vi "Main.vi"(11 "Module Admin":refnum<class "Delacor_lib_QMH_Cloneable Module Admin.lvclass">) -> ()   [LabVIEW 2025, in "USB IO.lvlib"]
doc: "This template is based off of the Queued Message Handler design pattern and the Queued Message Handler project template that ships with LabVIEW.\n\nThe main difference is that the queue is private to this module and communication between modules is performed via Broadcast and Request events.\n\nRequest events are wrapped in public API methods and are handled in the Event Handling Loop (EHL) of this VI. Any module can register for Broadcast events sent by this module. The EHL generates messages based on user interface actions.\n\nThe Message Handling Loop (MHL) processes messages generated by the EHL, or by other messages. The messages are string values, so new messages can be added easily to the Message Cases case structure in the MHL. Each message cluster can also provide an optional value for Message Data, which is a variant that can be converted to whatever message-specific data is required.\n_____\nBased on DQMH Dev Tools: Project Template 7.1.2.1547."
uses:
  USB IO.lvlib
  <vilib>/Delacor/Delacor QMH/Libraries/Message Queue_class/Delacor_lib_QMH_Message Queue.lvclass
  Module Data--cluster.ctl
  <vilib>/Utility/miscctls.llb/LVPointTypeDef.ctl
  <vilib>/Delacor/Delacor QMH/Libraries/Message Queue_class/Delacor_lib_QMH_Enqueue Message (Single).vi
  Stop Argument--cluster.ctl
  <vilib>/Delacor/Delacor QMH/Libraries/Cloneable Module Admin_class/Delacor_lib_QMH_Cloneable Module Admin.lvclass
  Display Lines (Reply Payload)--cluster.ctl
  Display Lines Argument--cluster.ctl
  Classes/USB IO generic/USB IO.lvclass
  select child (Reply Payload)--cluster.ctl
  Classes/Hardware Selection.ctl
  select child Argument--cluster.ctl
  Classes/Arduino Uno/Arduino Uno.lvclass
  Classes/USB-6000/USB-6000.lvclass
  read config (Reply Payload)--cluster.ctl
  read config Argument--cluster.ctl
  init device (Reply Payload)--cluster.ctl
  init device Argument--cluster.ctl
  stop device (Reply Payload)--cluster.ctl
  stop device Argument--cluster.ctl
  Controls/Numeric Voltage.ctl
  analog read (Reply Payload)--cluster.ctl
  analog read Argument--cluster.ctl
  digital write (Reply Payload)--cluster.ctl
  digital write Argument--cluster.ctl
  reconnect (Reply Payload)--cluster.ctl
  reconnect Argument--cluster.ctl
  C:/Users/grove/Desktop/LabVIEW/Git/atp-station/Libraries/USB IO/Classes/USB IO generic/USB IO.lvclass
  C:/Users/grove/Desktop/LabVIEW/Git/atp-station/Libraries/USB IO/Classes/USB-6000/USB-6000.lvclass
  C:/Users/grove/Desktop/LabVIEW/Git/atp-station/Libraries/USB IO/Classes/Arduino Uno/Arduino Uno.lvclass
panel:
  out "error out":errorcluster
  out "Status":string
  in  "Simulate EHL Error":bool
  in  "Simulate MHL Error":bool
  # "Other processes communicate with this Module via its Public API (wrappers for its Request Events).\n\nThis Module communicates with other processes via its Broadcast Events.\nAny process that wants to receive these messages can register for this module's Broadcast events."
  # "This template is for the DQMH framework. See the block diagram for more information on how to use this template."
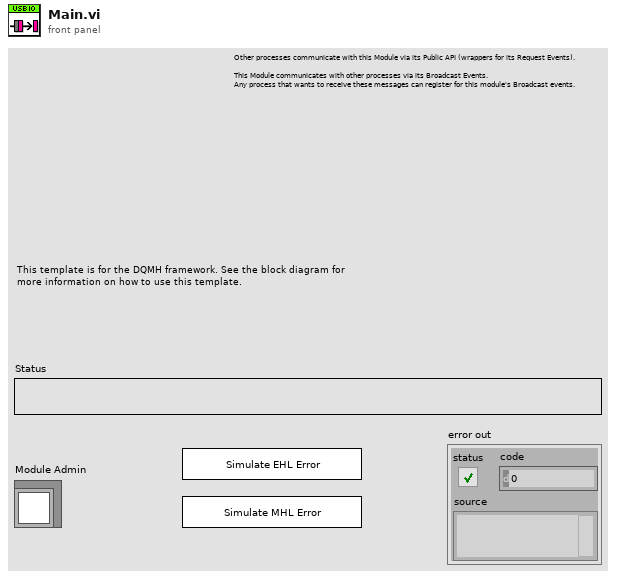
[diagram p1: front panel]
types:
  T1 = typedef "USB IO.lvlib/Request Events--cluster.ctl" = cluster{"Stop Module":refnum<user-event>, "Show Panel":refnum<user-event>, "Hide Panel":refnum<user-event>, "Show Diagram":refnum<user-event>, "Get Module Execution Status":refnum<user-event>, "Display Lines":refnum<user-event>, "select child":refnum<user-event>, "read config":refnum<user-event>, "init":refnum<user-event>, "init device":refnum<user-event>, "stop device":refnum<user-event>, "analog read":refnum<user-event>, "digital write":refnum<user-event>, "reconnect":refnum<user-event>}
  T2 = typedef "USB IO.lvlib/Module Data--cluster.ctl" = cluster{"Status":string, "USB IO.lvlib:USB IO.lvclass":refnum<class "USB IO.lvclass">}
  T3 = enum32{"invalid lock state", "Not Locked", "Locked (No Password)", "Password-protected"}
  T4 = typedef "USB IO.lvlib/Stop Argument--cluster.ctl" = cluster{"Module ID":i32, "Origin":string, "Exit via Stop Module Req?":bool, "Wait for Module to stop?":bool}
  T5 = typedef "USB IO.lvlib/Display Lines Argument--cluster.ctl" = cluster{"Module ID":i32, "Wait Notifier":refnum<notifier>, "wait for reply":bool}
  T6 = typedef "USB IO.lvlib/select child Argument--cluster.ctl" = cluster{"Module ID":i32, "Hardware":T7, "Wait Notifier":refnum<notifier>, "wait for reply":bool}
  T7 = typedef "Hardware Selection.ctl" = enum16{"Simulation", "USB-6000", "USB-6001", "Arduino Uno"}
  T8 = typedef "USB IO.lvlib/read config Argument--cluster.ctl" = cluster{"Module ID":i32, "Path":path, "Wait Notifier":refnum<notifier>, "wait for reply":bool}
  T9 = typedef "USB IO.lvlib/init device Argument--cluster.ctl" = cluster{"Module ID":i32, "Variant":variant, "Wait Notifier":refnum<notifier>, "wait for reply":bool}
  T10 = typedef "USB IO.lvlib/stop device Argument--cluster.ctl" = cluster{"Module ID":i32, "Wait Notifier":refnum<notifier>, "wait for reply":bool}
  T11 = typedef "USB IO.lvlib/analog read Argument--cluster.ctl" = cluster{"Module ID":i32, "Line":string, "Wait Notifier":refnum<notifier>, "wait for reply":bool}
  T12 = typedef "USB IO.lvlib/digital write Argument--cluster.ctl" = cluster{"Module ID":i32, "Line":string, "On/Off":bool, "Wait Notifier":refnum<notifier>, "wait for reply":bool}
  T13 = typedef "USB IO.lvlib/reconnect Argument--cluster.ctl" = cluster{"Module ID":i32, "Wait Notifier":refnum<notifier>, "wait for reply":bool}
  T14 = typedef "LVPointTypeDef.ctl" = cluster{"Horizontal":i16, "Vertical":i16}
  T15 = enum32{"Invalid", "Standard", "Closed", "Hidden", "Minimized", "Maximized"}
  T16 = typedef "USB IO.lvlib/Display Lines (Reply Payload)--cluster.ctl" = cluster{"Module ID":i32, "Lines":string[], "Values":i32[], "error":errorcluster}
  T17 = typedef "USB IO.lvlib/select child (Reply Payload)--cluster.ctl" = cluster{"Module ID":i32, "error":errorcluster}
  T18 = typedef "USB IO.lvlib/read config (Reply Payload)--cluster.ctl" = cluster{"Module ID":i32, "error":errorcluster}
  T19 = typedef "USB IO.lvlib/init device (Reply Payload)--cluster.ctl" = cluster{"Module ID":i32, "error":errorcluster}
  T20 = typedef "USB IO.lvlib/stop device (Reply Payload)--cluster.ctl" = cluster{"Module ID":i32, "error":errorcluster}
  T21 = typedef "USB IO.lvlib/analog read (Reply Payload)--cluster.ctl" = cluster{"Module ID":i32, "Voltage":T22, "error":errorcluster}
  T22 = typedef "Numeric Voltage.ctl" = dbl
  T23 = typedef "USB IO.lvlib/digital write (Reply Payload)--cluster.ctl" = cluster{"Module ID":i32, "error":errorcluster}
  T24 = typedef "USB IO.lvlib/reconnect (Reply Payload)--cluster.ctl" = cluster{"Module ID":i32, "error":errorcluster}
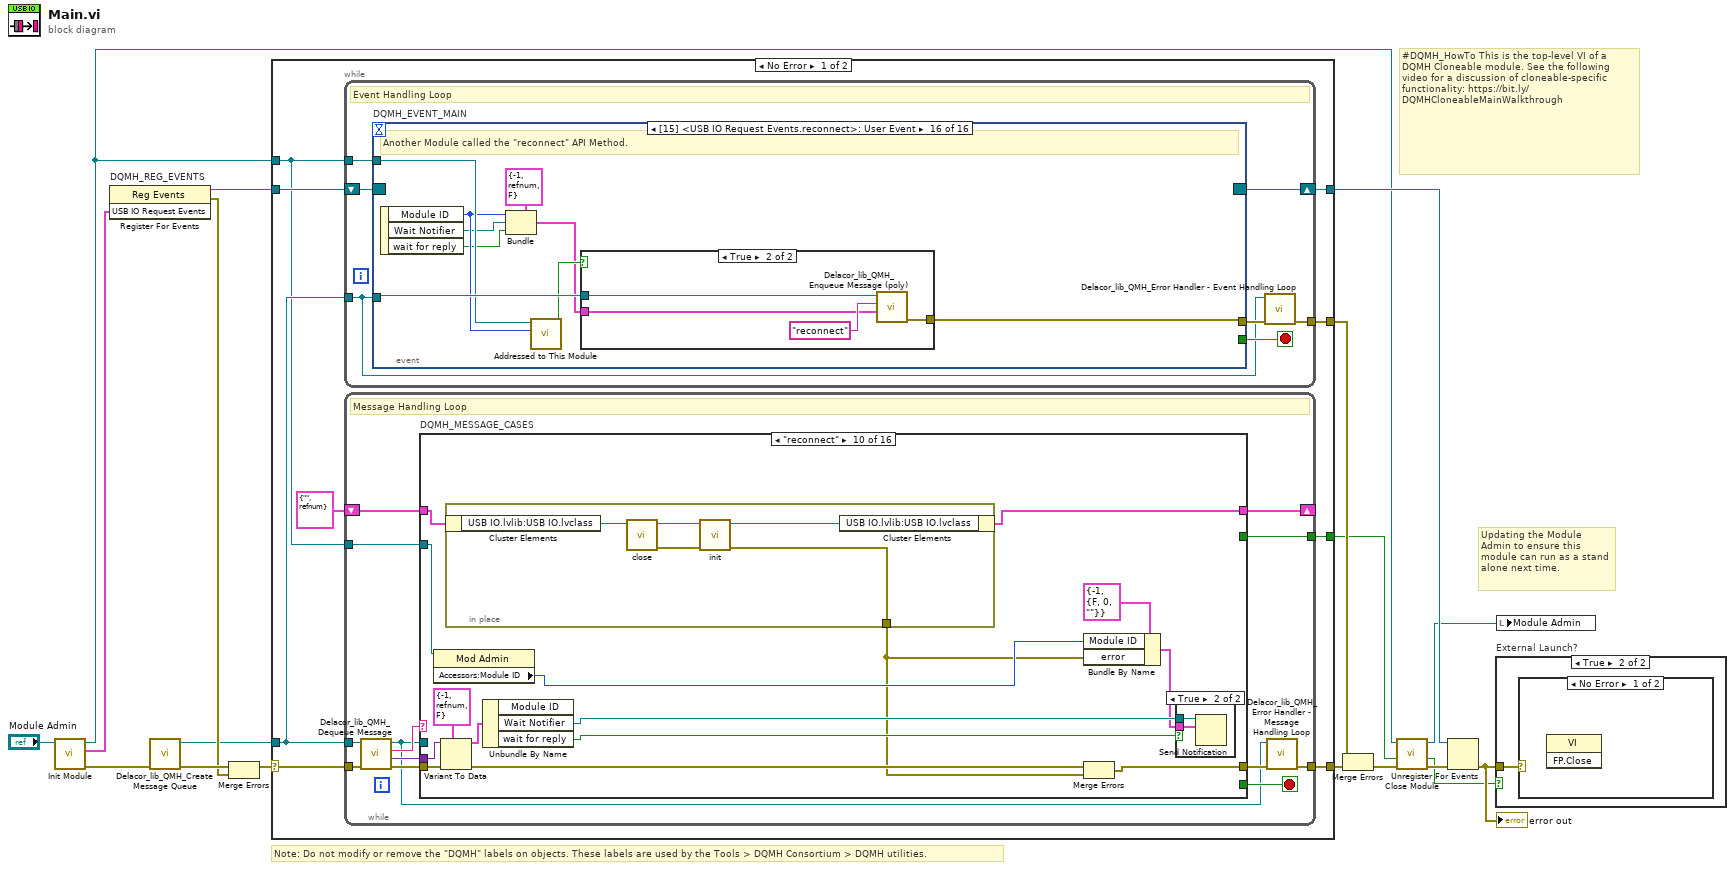
[diagram p0: block diagram]
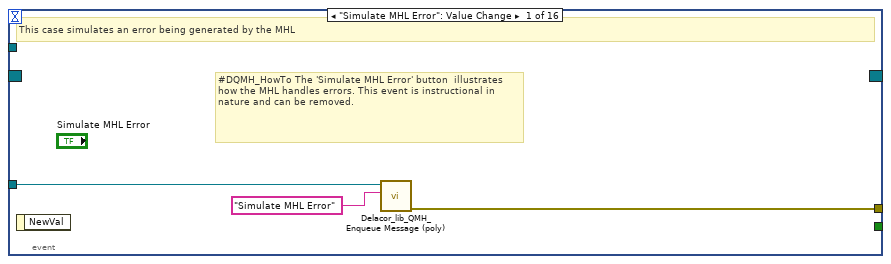
[diagram p2: hidden frame]
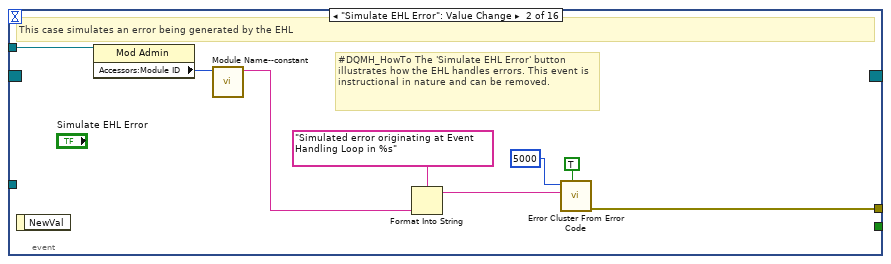
[diagram p3: hidden frame]
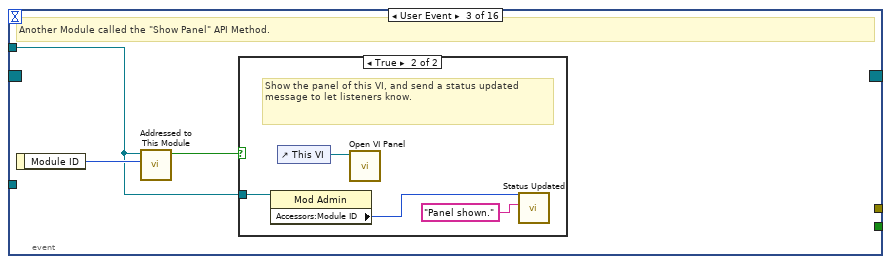
[diagram p4: hidden frame]
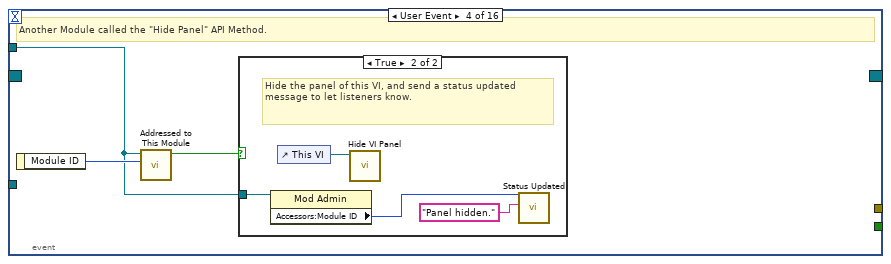
[diagram p6: hidden frame]
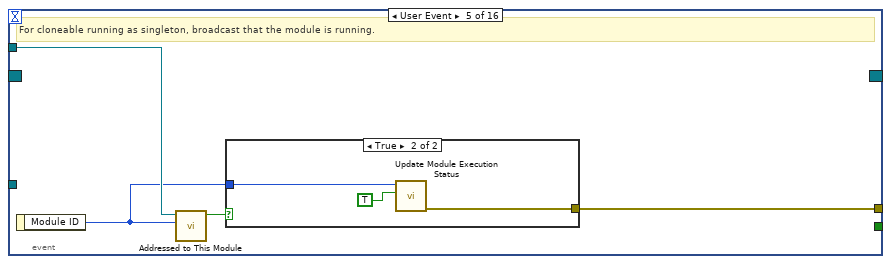
[diagram p8: hidden frame]
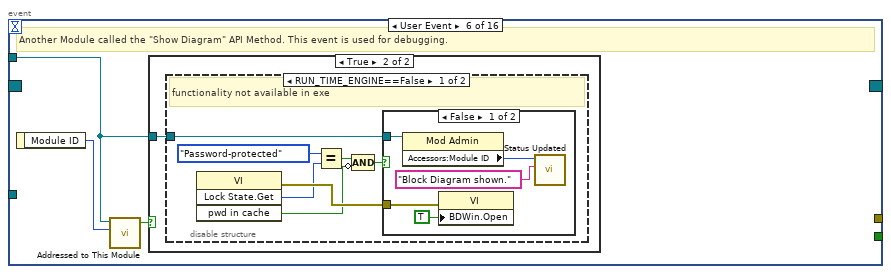
[diagram p10: hidden frame]
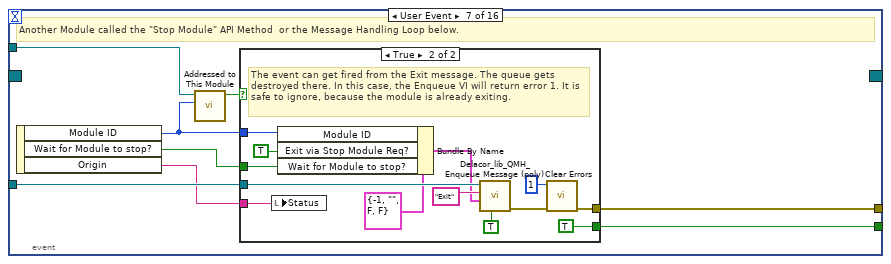
[diagram p14: hidden frame]
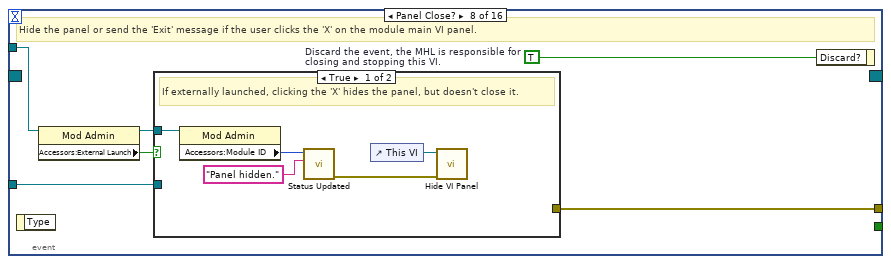
[diagram p16: hidden frame]
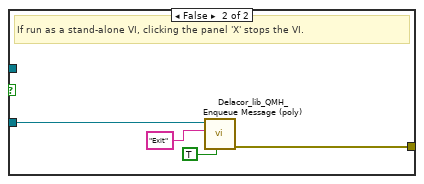
[diagram p17: hidden frame]
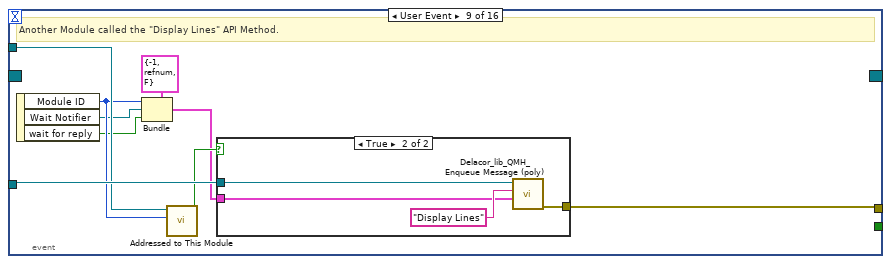
[diagram p18: hidden frame]
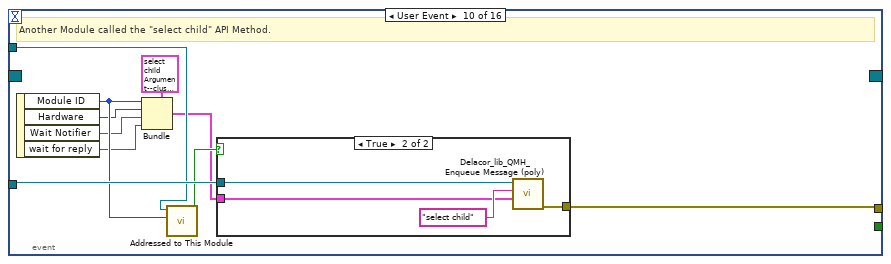
[diagram p20: hidden frame]
diagram:
  # "#DQMH_HowTo This is the top-level VI of a DQMH Cloneable module. See the following video for a discussion of cloneable-specific functionality: https://bit.ly/DQMHCloneableMainWalkthrough"
  # "Note: Do not modify or remove the \"DQMH\" labels on objects. These labels are used by the Tools > DQMH Consortium > DQMH utilities."
  # "Updating the Module Admin to ensure this module can run as a stand alone next time."
  n1 = call "Init Module.vi"("Cloneable Module Admin in"="Module Admin") -> ("error out"=w15:errorcluster, "USB IO Request Events"=w7:T1, "Cloneable Module Admin out"=w4:refnum<class "Delacor_lib_QMH_Cloneable Module Admin.lvclass">)  [unwired: 8 in]
  n2 = register-events "DQMH_REG_EVENTS"(w7) -> (reference out=w8:refnum<event-registration>, error out=w10:errorcluster)  [unwired: 2 in]
  n3 = call <vilib>:"Delacor_lib_QMH_Create Message Queue.vi"("error in"=w15) -> ("error out"=w12:errorcluster, "Message Queue"=w6:refnum<class "Delacor_lib_QMH_Message Queue.lvclass">)  [unwired: 9 in]
  n4 = Merge Errors(w12, w10) -> (w11:errorcluster)
  n5 = case shown="No Error" w11 {
    selector: w11 -> [w25 w517]
    tunnel: [w27 w516] -> w16
    tunnel: [w24 w515] -> w9
    tunnel: w8 -> [w22 w515]
    tunnel: w6 -> [w21 w508]
    tunnel: [w26 _] -> w17
    tunnel: w4 -> [w20 w511]
    tunnel: [w19 _] -> w2
    frame No Error {
      n6 = while {
        tunnel: w21 -> [w28]
        shift-right: [w31] -> w24
        shift-left: w22 -> [w32]
        tunnel: [w33] -> w26
        tunnel: w20 -> [w29]
        stop <- w30 stop-if-true
        # "Event Handling Loop"
        n7 = event "DQMH_EVENT_MAIN" shown="[15] <USB IO Request Events.reconnect>: User Event" {
          selector: w32 -> [_ _ _ _ _ _ _ _ _ _ _ _ _ _ _ _]
          dyn-events: [_ _ _ _ _ _ _ _ _ _ _ _ _ _ _ _] -> w31
          timeout: _ -> [_ _ _ _ _ _ _ _ _ _ _ _ _ _ _ _]
          tunnel: [_ _ _ _ _ _ w86 _ _ _ _ _ _ _ _ _] -> w30
          tunnel: w28 -> [w36 _ _ _ _ _ w89 w106 w127 w141 w155 w169 w182 w196 w211 w224]
          tunnel: [w37 w45 _ _ w63 _ w90 w109 w119 w132 w146 w160 w174 w187 w201 w216] -> w34
          tunnel: w29 -> [_ w44 w46 w53 w61 w67 w88 w107 w125 w139 w153 w167 w180 w194 w209 w222]
          event "Simulate MHL Error": Value Change {
            # "#DQMH_HowTo The 'Simulate MHL Error' button  illustrates how the MHL handles errors. This event is instructional in nature and can be removed."
            # "This case simulates an error being generated by the MHL"
            n8 = event-data() -> ()  [unwired: 1 in, 1 out]
            n9 = call-poly <vilib>:"Delacor_lib_QMH_Enqueue Message (poly).vi"("Message"="Simulate MHL Error", "Message Queue in"=w36) -> ("error out"=w37:errorcluster)  [unwired: 8 in, 1 out]
          }
          event "Simulate EHL Error": Value Change {
            # "#DQMH_HowTo The 'Simulate EHL Error' button  illustrates how the EHL handles errors. This event is instructional in nature and can be removed."
            # "This case simulates an error being generated by the EHL"
            n10 = event-data() -> ()  [unwired: 1 in, 1 out]
            n11 = property on="Property Node" class="Mod Admin"(reference=w44) -> ("Accessors:Module ID"=w43:i32)  [unwired: 1 in, 2 out]
            n12 = call "Module Name--constant.vi"("Module ID"=w43) -> ("Module Name"=w38:string)  [unwired: 10 in]
            n13 = Format Into String(format string="Simulated error originating at Event Handling Loop in %s", w38) -> (resulting string=w41:string)  [unwired: 2 in, 1 out]
            n14 = call <vilib>:"Error Cluster From Error Code.vi"("show call chain? (False)"=TRUE, "error message (\"\")"=w41, "error code (0)"=5000) -> ("error out"=w45:errorcluster)  [unwired: 6 in]
          }
          event User Event {
            # "Another Module called the \"Show Panel\" API Method."
            n15 = event-data() -> ("Module ID"=w47:i32)  [unwired: 1 in]
            n16 = call "Addressed to This Module.vi"("Module ID from Argument"=w47, "Module Admin"=w46) -> ("Addressed to this instance?"=w48:bool)  [unwired: 8 in, 1 out]
            n17 = case shown="True" w48 {
              tunnel: w46 -> [_ w50]
              frame False {
              }
              frame True {
                # "Show the panel of this VI, and send a status updated message to let listeners know."
                n18 = property on="Property Node" class="Mod Admin"(reference=w50) -> ("Accessors:Module ID"=w49:i32)  [unwired: 1 in, 2 out]
                n19 = control-ref of="This VI"() -> (w52:refnum<vi>)
                n20 = call "Open VI Panel.vi"("VI"=w52) -> ()  [unwired: 10 in, 1 out]
                n21 = call "Status Updated.vi"("Status"="Panel shown." ("format string"), "Module ID"=w49) -> ()  [unwired: 9 in, 1 out]
              }
            }
          }
          event User Event {
            # "Another Module called the \"Hide Panel\" API Method."
            n22 = event-data() -> ("Module ID"=w54:i32)  [unwired: 1 in]
            n23 = call "Addressed to This Module.vi"("Module ID from Argument"=w54, "Module Admin"=w53) -> ("Addressed to this instance?"=w55:bool)  [unwired: 8 in, 1 out]
            n24 = case shown="True" w55 {
              tunnel: w53 -> [_ w57]
              frame False {
              }
              frame True {
                # "Hide the panel of this VI, and send a status updated message to let listeners know."
                n25 = property on="Property Node" class="Mod Admin"(reference=w57) -> ("Accessors:Module ID"=w56:i32)  [unwired: 1 in, 2 out]
                n26 = control-ref of="This VI"() -> (w59:refnum<vi>)
                n27 = call "Hide VI Panel.vi"("VI"=w59) -> ()  [unwired: 10 in, 1 out]
                n28 = call "Status Updated.vi"("Status"="Panel hidden." ("format string"), "Module ID"=w56) -> ()  [unwired: 9 in, 1 out]
              }
            }
          }
          event User Event {
            # "For cloneable running as singleton, broadcast that the module is running."
            n29 = event-data() -> ("Module ID"=w60:i32)  [unwired: 1 in]
            n30 = call "Addressed to This Module.vi"("Module ID from Argument"=w60, "Module Admin"=w61) -> ("Addressed to this instance?"=w62:bool)  [unwired: 8 in, 1 out]
            n31 = case shown="True" w62 {
              tunnel: [_ w66] -> w63
              tunnel: w60 -> [_ w65]
              frame False {
              }
              frame True {
                n32 = call "Update Module Execution Status.vi"("Running?"=TRUE, "Module ID"=w65) -> ("error out"=w66:errorcluster)  [unwired: 9 in]
              }
            }
          }
          event User Event {
            # "Another Module called the \"Show Diagram\" API Method. This event is used for debugging."
            n33 = event-data() -> ("Module ID"=w68:i32)  [unwired: 1 in]
            n34 = call "Addressed to This Module.vi"("Module ID from Argument"=w68, "Module Admin"=w67) -> ("Addressed to this instance?"=w69:bool)  [unwired: 8 in, 1 out]
            n35 = case shown="True" w69 {
              tunnel: w67 -> [_ w70]
              frame False {
              }
              frame True {
                n36 = disable-structure shown="RUN_TIME_ENGINE==False" {
                  disable-tunnel: w70 -> [w71 _]
                  frame condition #0 (active) {
                    # "functionality not available in exe"
                    n37 = invoke on="Invoke Node" class="VI" method="Lock State.Get"() -> (error out=w77:errorcluster, "Get Lock State"=w76:T3, "pwd in cache"=w73:bool)  [unwired: 4 in, 1 out]
                    n38 = Equal?(x=T3."Password-protected", y=w76) -> (x = y?=w74:bool)
                    n39 = Compound Arithmetic op=AND(w74, invert w73) -> (w72:bool)
                    n40 = case shown="False" w72 {
                      tunnel: w77 -> [w82 _]
                      tunnel: w71 -> [w79 _]
                      frame False {
                        n41 = property on="Property Node" class="Mod Admin"(reference=w79) -> ("Accessors:Module ID"=w78:i32)  [unwired: 1 in, 2 out]
                        n42 = property on="Property Node" class="VI"(error in=w82, "BDWin.Open"=TRUE ("Block Diagram Window:Open")) -> ()  [unwired: 1 in, 2 out]
                        n43 = call "Status Updated.vi"("Status"="Block Diagram shown." ("format string"), "Module ID"=w78) -> ()  [unwired: 9 in, 1 out]
                      }
                      frame True {
                        # "Password-protected VI, and the password is not in the cache. Do not show the diagram."
                      }
                    }
                  }
                  frame condition #1 {
                  }
                }
              }
            }
          }
          event User Event {
            # "Another Module called the \"Stop Module\" API Method  or the Message Handling Loop below."
            n44 = event-data() -> ("Module ID"=w84:i32, "Wait for Module to stop?"=w85:bool, "Origin"=w83:string)  [unwired: 1 in]
            n45 = call "Addressed to This Module.vi"("Module ID from Argument"=w84, "Module Admin"=w88) -> ("Addressed to this instance?"=w87:bool)  [unwired: 8 in, 1 out]
            n46 = case shown="True" w87 {
              tunnel: [_ w102] -> w90
              tunnel: w89 -> [_ w98]
              tunnel: [_ TRUE] -> w86
              tunnel: w85 -> [_ w93]
              tunnel: w84 -> [_ w95]
              tunnel: w83 -> [_ w91]
              frame False {
              }
              frame True {
                # "The event can get fired from the Exit message. The queue gets destroyed there. In this case, the Enqueue VI will return error 1. It is safe to ignore, because the module is already exiting."
                n47 = local write "Status"(w91) -> ()
                n48 = Bundle By Name(cluster=T4 {"Module ID"=-1, "Origin"="", "Exit via Stop Module Req?"=FALSE, "Wait for Module to stop?"=FALSE} ("Stop Argument"), "Module ID"=w95, "Exit via Stop Module Req?"=TRUE, "Wait for Module to stop?"=w93) -> (w92:T4)
                n49 = call-poly <vilib>:"Delacor_lib_QMH_Enqueue Message (poly).vi"("Priority Message? (F)"=TRUE, "Message Data"=w92, "Message"="Exit", "Message Queue in"=w98) -> ("error out"=w103:errorcluster)  [unwired: 6 in, 1 out]
                n50 = call <vilib>:"Clear Errors.vi"("error in (no error)"=w103, "specific error code to clear (0: all)"=1) -> ("error out"=w102:errorcluster)  [unwired: 4 in, 1 out]
              }
            }
          }
          event Panel Close? {
            w108 = TRUE  # Discard the event, the MHL is responsible for closing and stopping this VI.
            # "Hide the panel or send the 'Exit' message if the user clicks the 'X' on the module main VI panel."
            n51 = event-data() -> ()  [unwired: 1 in, 1 out]
            n52 = property on="Property Node" class="Mod Admin"(reference=w107) -> (reference out=w104:refnum<class "Delacor_lib_QMH_Cloneable Module Admin.lvclass">, "Accessors:External Launch"=w105:bool)  [unwired: 1 in, 1 out]
            n53 = case shown="True" w105 {
              tunnel: w106 -> [_ w117]
              tunnel: [_ w118] -> w109
              tunnel: w104 -> [w112 _]
              frame True {
                # "If externally launched, clicking the 'X' hides the panel, but doesn't close it."
                n54 = property on="Property Node" class="Mod Admin"(reference=w112) -> ("Accessors:Module ID"=w111:i32)  [unwired: 1 in, 2 out]
                n55 = call "Status Updated.vi"("Status"="Panel hidden." ("format string"), "Module ID"=w111) -> ("error out"=w110:errorcluster)  [unwired: 9 in]
                n56 = control-ref of="This VI"() -> (w114:refnum<vi>)
                n57 = call "Hide VI Panel.vi"("error in"=w110, "VI"=w114) -> ()  [unwired: 9 in, 1 out]
              }
              frame False {
                # "If run as a stand-alone VI, clicking the panel 'X' stops the VI."
                n58 = call-poly <vilib>:"Delacor_lib_QMH_Enqueue Message (poly).vi"("Priority Message? (F)"=TRUE, "Message"="Exit", "Message Queue in"=w117) -> ("error out"=w118:errorcluster)  [unwired: 7 in, 1 out]
              }
            }
            n59 = event-data ("Event Filter Node")("Discard?"=w108) -> ()  [unwired: 1 in, 1 out]
          }
          event User Event {
            # "Another Module called the \"Display Lines\" API Method."
            n60 = event-data() -> ("Module ID"=w122:i32, "Wait Notifier"=w121:refnum<notifier>, "wait for reply"=w120:bool)  [unwired: 1 in]
            n61 = Bundle(cluster=T5 {"Module ID"=-1, "Wait Notifier"=refnum, "wait for reply"=FALSE} ("Display Lines Argument"), "Module ID"=w122, "Wait Notifier"=w121, "wait for reply"=w120) -> (w123:T5)
            n62 = call "Addressed to This Module.vi"("Module ID from Argument"=w122, "Module Admin"=w125) -> ("Addressed to this instance?"=w126:bool)  [unwired: 8 in, 1 out]
            n63 = case shown="True" w126 {
              tunnel: w127 -> [_ w131]
              tunnel: w123 -> [_ w129]
              tunnel: [_ w128] -> w119
              frame False {
              }
              frame True {
                n64 = call-poly <vilib>:"Delacor_lib_QMH_Enqueue Message (poly).vi"("Message Data"=w129, "Message"="Display Lines", "Message Queue in"=w131) -> ("error out"=w128:errorcluster)  [unwired: 7 in, 1 out]
              }
            }
          }
          event User Event {
            # "Another Module called the \"select child\" API Method."
            n65 = event-data() -> ("Module ID"=w136:i32, "Hardware"=w135:T7, "Wait Notifier"=w134:refnum<notifier>, "wait for reply"=w133:bool)  [unwired: 1 in]
            n66 = Bundle(cluster=T6 {"Module ID"=-1, "Hardware"=enum."USB-6000", "Wait Notifier"=refnum, "wait for reply"=FALSE} ("select child Argument"), "Module ID"=w136, "Hardware"=w135, "Wait Notifier"=w134, "wait for reply"=w133) -> (w137:T6)
            n67 = call "Addressed to This Module.vi"("Module ID from Argument"=w136, "Module Admin"=w139) -> ("Addressed to this instance?"=w140:bool)  [unwired: 8 in, 1 out]
            n68 = case shown="True" w140 {
              tunnel: w141 -> [_ w145]
              tunnel: w137 -> [_ w143]
              tunnel: [_ w142] -> w132
              frame False {
              }
              frame True {
                n69 = call-poly <vilib>:"Delacor_lib_QMH_Enqueue Message (poly).vi"("Message Data"=w143, "Message"="select child", "Message Queue in"=w145) -> ("error out"=w142:errorcluster)  [unwired: 7 in, 1 out]
              }
            }
          }
          event User Event {
            # "Another Module called the \"read config\" API Method."
            n70 = event-data() -> ("Module ID"=w150:i32, "Path"=w149:path, "Wait Notifier"=w148:refnum<notifier>, "wait for reply"=w147:bool)  [unwired: 1 in]
            n71 = Bundle(cluster=T8 {"Module ID"=-1, "Path"=path "", "Wait Notifier"=refnum, "wait for reply"=FALSE} ("read config Argument"), "Module ID"=w150, "Path"=w149, "Wait Notifier"=w148, "wait for reply"=w147) -> (w151:T8)
            n72 = call "Addressed to This Module.vi"("Module ID from Argument"=w150, "Module Admin"=w153) -> ("Addressed to this instance?"=w154:bool)  [unwired: 8 in, 1 out]
            n73 = case shown="True" w154 {
              tunnel: w155 -> [_ w159]
              tunnel: w151 -> [_ w157]
              tunnel: [_ w156] -> w146
              frame False {
              }
              frame True {
                n74 = call-poly <vilib>:"Delacor_lib_QMH_Enqueue Message (poly).vi"("Message Data"=w157, "Message"="read config", "Message Queue in"=w159) -> ("error out"=w156:errorcluster)  [unwired: 7 in, 1 out]
              }
            }
          }
          event User Event {
            # "Another Module called the \"init device\" API Method."
            n75 = event-data() -> ("Module ID"=w164:i32, "Variant"=w163:variant, "Wait Notifier"=w162:refnum<notifier>, "wait for reply"=w161:bool)  [unwired: 1 in]
            n76 = Bundle(cluster=T9 {"Module ID"=-1, "Variant"=variant, "Wait Notifier"=refnum, "wait for reply"=FALSE} ("init device Argument"), "Module ID"=w164, "Variant"=w163, "Wait Notifier"=w162, "wait for reply"=w161) -> (w165:T9)
            n77 = call "Addressed to This Module.vi"("Module ID from Argument"=w164, "Module Admin"=w167) -> ("Addressed to this instance?"=w168:bool)  [unwired: 8 in, 1 out]
            n78 = case shown="True" w168 {
              tunnel: w169 -> [_ w173]
              tunnel: w165 -> [_ w171]
              tunnel: [_ w170] -> w160
              frame False {
              }
              frame True {
                n79 = call-poly <vilib>:"Delacor_lib_QMH_Enqueue Message (poly).vi"("Message Data"=w171, "Message"="init device", "Message Queue in"=w173) -> ("error out"=w170:errorcluster)  [unwired: 7 in, 1 out]
              }
            }
          }
          event User Event {
            # "Another Module called the \"stop device\" API Method."
            n80 = event-data() -> ("Module ID"=w177:i32, "Wait Notifier"=w176:refnum<notifier>, "wait for reply"=w175:bool)  [unwired: 1 in]
            n81 = Bundle(cluster=T10 {"Module ID"=-1, "Wait Notifier"=refnum, "wait for reply"=FALSE} ("stop device Argument"), "Module ID"=w177, "Wait Notifier"=w176, "wait for reply"=w175) -> (w178:T10)
            n82 = call "Addressed to This Module.vi"("Module ID from Argument"=w177, "Module Admin"=w180) -> ("Addressed to this instance?"=w181:bool)  [unwired: 8 in, 1 out]
            n83 = case shown="True" w181 {
              tunnel: w182 -> [_ w186]
              tunnel: w178 -> [_ w184]
              tunnel: [_ w183] -> w174
              frame False {
              }
              frame True {
                n84 = call-poly <vilib>:"Delacor_lib_QMH_Enqueue Message (poly).vi"("Message Data"=w184, "Message"="stop device", "Message Queue in"=w186) -> ("error out"=w183:errorcluster)  [unwired: 7 in, 1 out]
              }
            }
          }
          event User Event {
            # "Another Module called the \"analog read\" API Method."
            n85 = event-data() -> ("Module ID"=w191:i32, "Line"=w190:string, "Wait Notifier"=w189:refnum<notifier>, "wait for reply"=w188:bool)  [unwired: 1 in]
            n86 = Bundle(cluster=T11 {"Module ID"=-1, "Line"="", "Wait Notifier"=refnum, "wait for reply"=FALSE} ("analog read Argument"), "Module ID"=w191, "Line"=w190, "Wait Notifier"=w189, "wait for reply"=w188) -> (w192:T11)
            n87 = call "Addressed to This Module.vi"("Module ID from Argument"=w191, "Module Admin"=w194) -> ("Addressed to this instance?"=w195:bool)  [unwired: 8 in, 1 out]
            n88 = case shown="True" w195 {
              tunnel: w196 -> [_ w200]
              tunnel: w192 -> [_ w198]
              tunnel: [_ w197] -> w187
              frame False {
              }
              frame True {
                n89 = call-poly <vilib>:"Delacor_lib_QMH_Enqueue Message (poly).vi"("Message Data"=w198, "Message"="analog read", "Message Queue in"=w200) -> ("error out"=w197:errorcluster)  [unwired: 7 in, 1 out]
              }
            }
          }
          event User Event {
            # "Another Module called the \"digital write\" API Method."
            n90 = event-data() -> ("Module ID"=w206:i32, "Line"=w205:string, "On/Off"=w204:bool, "Wait Notifier"=w203:refnum<notifier>, "wait for reply"=w202:bool)  [unwired: 1 in]
            n91 = Bundle(cluster=T12 {"Module ID"=-1, "Line"="", "On/Off"=FALSE, "Wait Notifier"=refnum, "wait for reply"=FALSE} ("digital write Argument"), "Module ID"=w206, "Line"=w205, "On/Off"=w204, "Wait Notifier"=w203, "wait for reply"=w202) -> (w207:T12)
            n92 = call "Addressed to This Module.vi"("Module ID from Argument"=w206, "Module Admin"=w209) -> ("Addressed to this instance?"=w210:bool)  [unwired: 8 in, 1 out]
            n93 = case shown="True" w210 {
              tunnel: w211 -> [_ w215]
              tunnel: w207 -> [_ w213]
              tunnel: [_ w212] -> w201
              frame False {
              }
              frame True {
                n94 = call-poly <vilib>:"Delacor_lib_QMH_Enqueue Message (poly).vi"("Message Data"=w213, "Message"="digital write", "Message Queue in"=w215) -> ("error out"=w212:errorcluster)  [unwired: 7 in, 1 out]
              }
            }
          }
          event User Event {
            # "Another Module called the \"reconnect\" API Method."
            n95 = event-data() -> ("Module ID"=w219:i32, "Wait Notifier"=w218:refnum<notifier>, "wait for reply"=w217:bool)  [unwired: 1 in]
            n96 = Bundle(cluster=T13 {"Module ID"=-1, "Wait Notifier"=refnum, "wait for reply"=FALSE} ("reconnect Argument"), "Module ID"=w219, "Wait Notifier"=w218, "wait for reply"=w217) -> (w220:T13)
            n97 = call "Addressed to This Module.vi"("Module ID from Argument"=w219, "Module Admin"=w222) -> ("Addressed to this instance?"=w223:bool)  [unwired: 8 in, 1 out]
            n98 = case shown="True" w223 {
              tunnel: w224 -> [_ w228]
              tunnel: w220 -> [_ w226]
              tunnel: [_ w225] -> w216
              frame False {
              }
              frame True {
                n99 = call-poly <vilib>:"Delacor_lib_QMH_Enqueue Message (poly).vi"("Message Data"=w226, "Message"="reconnect", "Message Queue in"=w228) -> ("error out"=w225:errorcluster)  [unwired: 7 in, 1 out]
              }
            }
          }
        }
        n100 = call-dynamic "Delacor_lib_QMH_Error Handler - Event Handling Loop.vi"("error in"=w34, "Message Queue in"=w28) -> ("dup error in"=w33:errorcluster)  [unwired: 8 in, 1 out]
      }
      n101 = while {
        tunnel: w21 -> [w229]
        shift-right: [w236] -> _
        shift-left: T2 {"Status"="", "USB IO.lvlib:USB IO.lvclass"=refnum} ("Data Cluster") -> [w237]
        tunnel: w25 -> [w240]
        tunnel: [w238] -> w27
        tunnel: w20 -> [w231]
        tunnel: [w230] -> w19
        stop <- w235 stop-if-true
        # "Message Handling Loop"
        n102 = call-dynamic "Delacor_lib_QMH_Dequeue Message.vi"("error in"=w240, "Message Queue in"=w229) -> ("error out"=w239:errorcluster, "Message Data"=w233:variant, "Message"=w234:string, "Message Queue out"=w232:refnum<class "Delacor_lib_QMH_Message Queue.lvclass">)  [unwired: 6 in]
        n103 = case "DQMH_MESSAGE_CASES" shown="\"reconnect\"" w234 {
          selector: w234 -> [_ _ _ _ _ _ _ _ _ _ _ _ _ _ _ w497]
          tunnel: w232 -> [_ _ _ _ _ _ _ _ _ _ _ _ w452 _ w489 _]
          tunnel: w239 -> [w260 w264 w281 w304 w326 w348 w369 w391 w415 w437 w447 w449 w461 w478 w495 w506]
          tunnel: [w258 w264 w272 w295 w317 w339 w360 w382 w406 w428 w446 w449 w457 w477 w490 w507] -> w241
          tunnel: w237 -> [w251 w263 w268 w292 w314 w336 w357 w379 w403 w425 w445 w448 w456 w475 w488 w504]
          tunnel: [w250 w263 w269 w290 w313 w335 w356 w378 w402 w424 w445 w448 w456 w475 w488 w504] -> w236
          tunnel: [_ _ _ _ _ _ _ _ _ _ _ _ _ _ w487 _] -> w235
          tunnel: w233 -> [_ _ w279 w302 w324 w346 w367 w389 w413 w435 _ _ w455 _ w485 _]
          tunnel: w231 -> [w246 _ w270 w293 w315 w337 w358 w380 w404 w426 _ _ w454 w473 w480 w503]
          tunnel: [_ _ _ _ _ _ _ _ _ _ _ _ _ _ w483 _] -> w230
          frame "Initialize" {
            w243 = "Initial Message" ("Initial Message")
            # "#DQMH_CodeNeeded - Initialize the appearance of the front panel."
            # "#DQMH_CodeNeeded - Initialize your state data here."
            # "Initialize - Any operation that needs to be done before the module can receive messages. Synchronize Caller Events.vi will inform Start Module.vi that the module has launched and is ready to receive messages. Module Did Init.vi will broadcast that the module initialized."
            n104 = call "Synchronize Caller Events.vi"("error in"=w260, "Module Admin"=w246) -> ("error out"=w259:errorcluster, "Module Admin out"=w245:refnum<class "Delacor_lib_QMH_Cloneable Module Admin.lvclass">)  [unwired: 8 in]
            n105 = property on="Property Node" class="Mod Admin"(reference=w245) -> ("Accessors:Module ID"=w242:i32, "Accessors:External Launch"=w247:bool)  [unwired: 1 in, 2 out]
            n106 = call "Module Name--constant.vi"("Module ID"=w242) -> ("Module Name"=w255:string)  [unwired: 10 in]
            n107 = property on="Property Node" class="VI"("Front Panel.Title"=w255) -> (reference out=w257:refnum<vi>, error out=w262:errorcluster)  [unwired: 2 in]
            n108 = Select(t=T15."Hidden" ("State"), s=w247, f=T15."Standard" ("State")) -> (s? t:f=w252:T15)
            n109 = invoke on="Invoke Node" class="VI" method="FP.Open"(reference=w257, error in=w262, "State"=w252) -> (reference out=w256:refnum<vi>, error out=w261:errorcluster)  [unwired: 2 in, 3 out]
            n110 = Bundle By Name(cluster=w251, "Status"=w243) -> (w250:T2)
            n111 = invoke on="Invoke Node" class="VI" method="FP.Center"(reference=w256, error in=w261) -> ()  [unwired: 1 in, 3 out]
            n112 = property on="Pane" class="Pane"("Origin"=T14 {"Horizontal"=0, "Vertical"=0}) -> ()  [unwired: 2 in, 2 out]
            n113 = call "Module Name--constant.vi"("Module ID"=w242) -> ("Module Name"=w248:string)  [unwired: 10 in]
            n114 = call "Module Did Init.vi"("error in"=w259, "Initialized?"=TRUE, "Origin"=w248, "Module ID"=w242) -> ("error out"=w258:errorcluster)  [unwired: 7 in]
            "Status" <- w243
          }
          frame "---Module Specific---" {
            # "Separator -- The following cases handle messages specific to this Module."
          }
          frame "Display Lines" {
            n115 = property class="Mod Admin"(reference=w270) -> ("Accessors:Module ID"=w271:i32)  [unwired: 1 in, 2 out]
            n116 = Variant To Data(error in=w281, type=T5 {"Module ID"=-1, "Wait Notifier"=refnum, "wait for reply"=FALSE} ("Display Lines Argument"), Variant=w279) -> (data=w277:T5, error out=w280:errorcluster)
            n117 = in-place {
              in-place-border: [w284] -> w267
              in-place-border: [w283] -> w266
              in-place-border: [w282] -> w265
              n118 = in-place-cluster #1(w268) -> ("USB IO.lvlib:USB IO.lvclass"=w286:refnum<class "USB IO.lvclass">)
              n119 = call-dynamic "display lines.vi"("USB IO in"=w286) -> ("error out"=w282:errorcluster, "Values"=w283:i32[], "Lines"=w284:string[], "USB IO out"=w285:refnum<class "USB IO.lvclass">)  [unwired: 7 in]
              n120 = in-place-cluster #1("USB IO.lvlib:USB IO.lvclass"=w285) -> (w269:T2)
            }
            n121 = Unbundle By Name(w277) -> ("Wait Notifier"=w276:refnum<notifier>, "wait for reply"=w275:bool)  [unwired: 1 out]
            n122 = Bundle By Name(cluster=T16 {"Module ID"=-1, "Lines"=[], "Values"=[], "error"={"status"=FALSE, "code"=0, "source"=""}} ("Display Lines (Reply Payload)"), "Module ID"=w271, "Lines"=w267, "Values"=w266, "error"=w265) -> (w274:T16)
            n123 = Merge Errors(w280, w265) -> (w272:errorcluster)
            n124 = case "DQMH_FIRE_NOTIFIER" shown="True" w275 {
              tunnel: w276 -> [_ w288]
              tunnel: w274 -> [_ w287]
              frame False {
              }
              frame True {
                n125 = Send Notification(notification=w287, notifier=w288) -> ()  [unwired: 1 in, 2 out]
              }
            }
          }
          frame "select child" {
            w289 = errorcluster {"status"=FALSE, "code"=0, "source"=""} ("error")
            n126 = property class="Mod Admin"(reference=w293) -> ("Accessors:Module ID"=w294:i32)  [unwired: 1 in, 2 out]
            n127 = Variant To Data(error in=w304, type=T6 {"Module ID"=-1, "Hardware"=enum."USB-6000", "Wait Notifier"=refnum, "wait for reply"=FALSE} ("select child Argument"), Variant=w302) -> (data=w300:T6, error out=w303:errorcluster)
            n128 = Unbundle By Name(w300) -> ("Hardware"=w291:T7, "Wait Notifier"=w299:refnum<notifier>, "wait for reply"=w298:bool)  [unwired: 1 out]
            n129 = in-place {
              in-place-border: w291 -> [w306]
              n130 = in-place-cluster #2(w292) -> ()  [unwired: 1 out]
              n131 = case shown="\"Arduino Uno\"" w306 {
                tunnel: [refnum<class "USB-6000.lvclass"> refnum ("USB IO.lvlib:USB-6000.lvclass") refnum<class "Arduino Uno.lvclass"> refnum ("USB IO.lvlib:Arduino Uno.lvclass")] -> w305
                frame "USB-6000", Default {
                }
                frame "Arduino Uno" {
                }
              }
              n132 = in-place-cluster #2("USB IO.lvlib:USB IO.lvclass"=w305) -> (w290:T2)
            }
            n133 = Bundle By Name(cluster=T17 {"Module ID"=-1, "error"={"status"=FALSE, "code"=0, "source"=""}} ("select child (Reply Payload)"), "Module ID"=w294, "error"=w289) -> (w297:T17)
            n134 = Merge Errors(w303, w289) -> (w295:errorcluster)
            n135 = case "DQMH_FIRE_NOTIFIER" shown="True" w298 {
              tunnel: w299 -> [_ w310]
              tunnel: w297 -> [_ w309]
              frame False {
              }
              frame True {
                n136 = Send Notification(notification=w309, notifier=w310) -> ()  [unwired: 1 in, 2 out]
              }
            }
          }
          frame "read config" {
            n137 = property class="Mod Admin"(reference=w315) -> ("Accessors:Module ID"=w316:i32)  [unwired: 1 in, 2 out]
            n138 = Variant To Data(error in=w326, type=T8 {"Module ID"=-1, "Path"=path "", "Wait Notifier"=refnum, "wait for reply"=FALSE} ("read config Argument"), Variant=w324) -> (data=w322:T8, error out=w325:errorcluster)
            n139 = Unbundle By Name(w322) -> ("Path"=w312:path, "Wait Notifier"=w321:refnum<notifier>, "wait for reply"=w320:bool)  [unwired: 1 out]
            n140 = in-place {
              in-place-border: w312 -> [w328]
              in-place-border: [w327] -> w311
              n141 = in-place-cluster #3(w314) -> ("USB IO.lvlib:USB IO.lvclass"=w330:refnum<class "USB IO.lvclass">)
              n142 = call-dynamic "read config.vi"("Path"=w328, "USB IO in"=w330) -> ("error out"=w327:errorcluster, "USB IO out"=w329:refnum<class "USB IO.lvclass">)  [unwired: 8 in]
              n143 = in-place-cluster #3("USB IO.lvlib:USB IO.lvclass"=w329) -> (w313:T2)
            }
            n144 = Bundle By Name(cluster=T18 {"Module ID"=-1, "error"={"status"=FALSE, "code"=0, "source"=""}} ("read config (Reply Payload)"), "Module ID"=w316, "error"=w311) -> (w319:T18)
            n145 = Merge Errors(w325, w311) -> (w317:errorcluster)
            n146 = case "DQMH_FIRE_NOTIFIER" shown="True" w320 {
              tunnel: w321 -> [_ w332]
              tunnel: w319 -> [_ w331]
              frame False {
              }
              frame True {
                n147 = Send Notification(notification=w331, notifier=w332) -> ()  [unwired: 1 in, 2 out]
              }
            }
          }
          frame "init device" {
            n148 = property class="Mod Admin"(reference=w337) -> ("Accessors:Module ID"=w338:i32)  [unwired: 1 in, 2 out]
            n149 = Variant To Data(error in=w348, type=T9 {"Module ID"=-1, "Variant"=variant, "Wait Notifier"=refnum, "wait for reply"=FALSE} ("init device Argument"), Variant=w346) -> (data=w344:T9, error out=w347:errorcluster)
            n150 = Unbundle By Name(w344) -> ("Variant"=w333:variant, "Wait Notifier"=w343:refnum<notifier>, "wait for reply"=w342:bool)  [unwired: 1 out]
            n151 = in-place {
              in-place-border: [w350] -> w334
              in-place-border: w333 -> [w349]
              n152 = in-place-cluster #4(w336) -> ("USB IO.lvlib:USB IO.lvclass"=w352:refnum<class "USB IO.lvclass">)
              n153 = call-dynamic "init.vi"("Variant"=w349, "USB IO in"=w352) -> ("error out"=w350:errorcluster, "USB IO out"=w351:refnum<class "USB IO.lvclass">)  [unwired: 8 in]
              n154 = in-place-cluster #4("USB IO.lvlib:USB IO.lvclass"=w351) -> (w335:T2)
            }
            n155 = Bundle By Name(cluster=T19 {"Module ID"=-1, "error"={"status"=FALSE, "code"=0, "source"=""}} ("init device (Reply Payload)"), "Module ID"=w338, "error"=w334) -> (w341:T19)
            n156 = Merge Errors(w347, w334) -> (w339:errorcluster)
            n157 = case "DQMH_FIRE_NOTIFIER" shown="True" w342 {
              tunnel: w343 -> [_ w354]
              tunnel: w341 -> [_ w353]
              frame False {
              }
              frame True {
                n158 = Send Notification(notification=w353, notifier=w354) -> ()  [unwired: 1 in, 2 out]
              }
            }
          }
          frame "stop device" {
            n159 = property class="Mod Admin"(reference=w358) -> ("Accessors:Module ID"=w359:i32)  [unwired: 1 in, 2 out]
            n160 = Variant To Data(error in=w369, type=T10 {"Module ID"=-1, "Wait Notifier"=refnum, "wait for reply"=FALSE} ("stop device Argument"), Variant=w367) -> (data=w365:T10, error out=w368:errorcluster)
            n161 = in-place {
              in-place-border: [w370] -> w355
              n162 = in-place-cluster #5(w357) -> ("USB IO.lvlib:USB IO.lvclass"=w372:refnum<class "USB IO.lvclass">)
              n163 = call-dynamic "close.vi"("USB IO in"=w372) -> ("error out"=w370:errorcluster, "USB IO out"=w371:refnum<class "USB IO.lvclass">)  [unwired: 9 in]
              n164 = in-place-cluster #5("USB IO.lvlib:USB IO.lvclass"=w371) -> (w356:T2)
            }
            n165 = Unbundle By Name(w365) -> ("Wait Notifier"=w364:refnum<notifier>, "wait for reply"=w363:bool)  [unwired: 1 out]
            n166 = Bundle By Name(cluster=T20 {"Module ID"=-1, "error"={"status"=FALSE, "code"=0, "source"=""}} ("stop device (Reply Payload)"), "Module ID"=w359, "error"=w355) -> (w362:T20)
            n167 = Merge Errors(w368, w355) -> (w360:errorcluster)
            n168 = case "DQMH_FIRE_NOTIFIER" shown="True" w363 {
              tunnel: w364 -> [_ w374]
              tunnel: w362 -> [_ w373]
              frame False {
              }
              frame True {
                n169 = Send Notification(notification=w373, notifier=w374) -> ()  [unwired: 1 in, 2 out]
              }
            }
          }
          frame "analog read" {
            n170 = property class="Mod Admin"(reference=w380) -> ("Accessors:Module ID"=w381:i32)  [unwired: 1 in, 2 out]
            n171 = Variant To Data(error in=w391, type=T11 {"Module ID"=-1, "Line"="", "Wait Notifier"=refnum, "wait for reply"=FALSE} ("analog read Argument"), Variant=w389) -> (data=w387:T11, error out=w390:errorcluster)
            n172 = Unbundle By Name(w387) -> ("Line"=w377:string, "Wait Notifier"=w386:refnum<notifier>, "wait for reply"=w385:bool)  [unwired: 1 out]
            n173 = in-place {
              in-place-border: w377 -> [w394]
              in-place-border: [w393] -> w376
              in-place-border: [w392] -> w375
              n174 = in-place-cluster #6(w379) -> ("USB IO.lvlib:USB IO.lvclass"=w396:refnum<class "USB IO.lvclass">)
              n175 = call-dynamic "analog read.vi"("Line"=w394, "USB IO in"=w396) -> ("error out"=w392:errorcluster, "Voltage"=w393:dbl, "USB IO out"=w395:refnum<class "USB IO.lvclass">)  [unwired: 7 in]
              n176 = in-place-cluster #6("USB IO.lvlib:USB IO.lvclass"=w395) -> (w378:T2)
            }
            n177 = Bundle By Name(cluster=T21 {"Module ID"=-1, "Voltage"=0.0, "error"={"status"=FALSE, "code"=0, "source"=""}} ("analog read (Reply Payload)"), "Module ID"=w381, "Voltage"=w376, "error"=w375) -> (w384:T21)
            n178 = Merge Errors(w390, w375) -> (w382:errorcluster)
            n179 = case "DQMH_FIRE_NOTIFIER" shown="True" w385 {
              tunnel: w386 -> [_ w398]
              tunnel: w384 -> [_ w397]
              frame False {
              }
              frame True {
                n180 = Send Notification(notification=w397, notifier=w398) -> ()  [unwired: 1 in, 2 out]
              }
            }
          }
          frame "digital write" {
            n181 = Variant To Data(error in=w415, type=T12 {"Module ID"=-1, "Line"="", "On/Off"=FALSE, "Wait Notifier"=refnum, "wait for reply"=FALSE} ("digital write Argument"), Variant=w413) -> (data=w411:T12, error out=w414:errorcluster)
            n182 = property class="Mod Admin"(reference=w404) -> ("Accessors:Module ID"=w405:i32)  [unwired: 1 in, 2 out]
            n183 = Unbundle By Name(w411) -> ("Line"=w400:string, "On/Off"=w399:bool, "Wait Notifier"=w410:refnum<notifier>, "wait for reply"=w409:bool)  [unwired: 1 out]
            n184 = in-place {
              in-place-border: [w419] -> w401
              in-place-border: w400 -> [w418]
              in-place-border: w399 -> [w417]
              n185 = in-place-cluster #7(w403) -> ("USB IO.lvlib:USB IO.lvclass"=w416:refnum<class "USB IO.lvclass">)
              n186 = call-dynamic "digital write.vi"("On/Off"=w417, "Line"=w418, "USB IO in"=w416) -> ("error out"=w419:errorcluster, "USB IO out"=w420:refnum<class "USB IO.lvclass">)  [unwired: 7 in]
              n187 = in-place-cluster #7("USB IO.lvlib:USB IO.lvclass"=w420) -> (w402:T2)
            }
            n188 = Bundle By Name(cluster=T23 {"Module ID"=-1, "error"={"status"=FALSE, "code"=0, "source"=""}} ("digital write (Reply Payload)"), "Module ID"=w405, "error"=w401) -> (w408:T23)
            n189 = Merge Errors(w414, w401) -> (w406:errorcluster)
            n190 = case "DQMH_FIRE_NOTIFIER" shown="True" w409 {
              tunnel: w410 -> [_ w422]
              tunnel: w408 -> [_ w421]
              frame False {
              }
              frame True {
                n191 = Send Notification(notification=w421, notifier=w422) -> ()  [unwired: 1 in, 2 out]
              }
            }
          }
          frame "reconnect" {
            n192 = property class="Mod Admin"(reference=w426) -> ("Accessors:Module ID"=w427:i32)  [unwired: 1 in, 2 out]
            n193 = Variant To Data(error in=w437, type=T13 {"Module ID"=-1, "Wait Notifier"=refnum, "wait for reply"=FALSE} ("reconnect Argument"), Variant=w435) -> (data=w433:T13, error out=w436:errorcluster)
            n194 = in-place {
              in-place-border: [w438] -> w423
              n195 = in-place-cluster #8(w425) -> ("USB IO.lvlib:USB IO.lvclass"=w440:refnum<class "USB IO.lvclass">)
              n196 = call-dynamic "close.vi"("USB IO in"=w440) -> ("error out"=w439:errorcluster, "USB IO out"=w441:refnum<class "USB IO.lvclass">)  [unwired: 9 in]
              n197 = call-dynamic "init.vi"("error in (no error)"=w439, "USB IO in"=w441) -> ("error out"=w438:errorcluster, "USB IO out"=w442:refnum<class "USB IO.lvclass">)  [unwired: 8 in]
              n198 = in-place-cluster #8("USB IO.lvlib:USB IO.lvclass"=w442) -> (w424:T2)
            }
            n199 = Unbundle By Name(w433) -> ("Wait Notifier"=w432:refnum<notifier>, "wait for reply"=w431:bool)  [unwired: 1 out]
            n200 = Bundle By Name(cluster=T24 {"Module ID"=-1, "error"={"status"=FALSE, "code"=0, "source"=""}} ("reconnect (Reply Payload)"), "Module ID"=w427, "error"=w423) -> (w430:T24)
            n201 = Merge Errors(w436, w423) -> (w428:errorcluster)
            n202 = case "DQMH_FIRE_NOTIFIER" shown="True" w431 {
              tunnel: w432 -> [_ w444]
              tunnel: w430 -> [_ w443]
              frame False {
              }
              frame True {
                n203 = Send Notification(notification=w443, notifier=w444) -> ()  [unwired: 1 in, 2 out]
              }
            }
          }
          frame "---Copy This Frame---" {
            # "Duplicate this frame when creating new messages.  Change this comment in the duplicated frame to describe this message."
            n204 = Merge Errors(w447) -> (w446:errorcluster)
          }
          frame "---Exit and Error Handling---" {
            # "Separator - the following cases handle errors and exit messages."
          }
          frame "Error" {
            # "#DQMH_CodeRecommended - If the module is running in standalone mode (External Launch = FALSE), this code will pop up an error dialog and call the 'Exit' message if an error occurs. Add more fine-grained error management here."
            # "Error - Check the error message data and respond accordingly. This message is sent by the \"Error Handler\" VIs at the end of each loop in this application."
            n205 = property on="Property Node" class="Mod Admin"(reference=w454) -> ("Accessors:External Launch"=w453:bool, "Accessors:Module ID"=w451:i32)  [unwired: 1 in, 2 out]
            n206 = Variant To Data(error in=w461, type=errorcluster {"status"=FALSE, "code"=0, "source"=""} ("error constant"), Variant=w455) -> (data=w450:errorcluster, error out=w459:errorcluster)
            n207 = local write "error out"(w450) -> ()
            n208 = call "Error Reported.vi"("Error"=w450, "Module ID"=w451) -> ()  [unwired: 9 in, 1 out]
            n209 = case shown="False" w453 {
              tunnel: [w466 _] -> w458
              tunnel: w452 -> [w464 _]
              tunnel: w450 -> [w465 _]
              frame False {
                n210 = disable-structure shown="Default" {
                  disable-tunnel: w465 -> [w467 _]
                  frame condition #0 (active) {
                    # "If the module is running standalone, then pop up an error dialog and call the \"Exit\" message."
                    n211 = call <vilib>:"Simple Error Handler.vi"("error in (no error)"=w467) -> ()  [unwired: 4 in, 5 out]
                  }
                  frame condition #1 {
                    # "To prevent the Simple Error Handler VI from being loaded (e.g. when deploying to a Real-Time target), add the Conditional Disable Symbol \"DQMH_Disable_SEH\" to your project and set it to TRUE."
                  }
                }
                n212 = call-poly <vilib>:"Delacor_lib_QMH_Enqueue Message (poly).vi"("Priority Message? (F)"=TRUE, "Message"="Exit", "Message Queue in"=w464) -> ("error out"=w466:errorcluster)  [unwired: 7 in, 1 out]
              }
              frame True {
                # "If the module was launched externally, calling the Error Reported broadcast VI is the only action performed by the \"Error\" message. The module's caller can then process the error appropriately."
              }
            }
            n213 = Merge Errors(w459, w458) -> (w457:errorcluster)
          }
          frame "Simulate MHL Error" {
            # "#DQMH_HowTo The 'Simulate MHL Error' button  illustrates how the MHL handles errors. This event is instructional in nature and can be removed."
            # "Simulate an error occurring at the MHL"
            n214 = property on="Property Node" class="Mod Admin"(reference=w473) -> ("Accessors:Module ID"=w474:i32)  [unwired: 1 in, 2 out]
            n215 = call "Module Name--constant.vi"("Module ID"=w474) -> ("Module Name"=w469:string)  [unwired: 10 in]
            n216 = Format Into String(format string="Simulated error originating at Message Handling Loop in %s", w469) -> (resulting string=w470:string)  [unwired: 2 in, 1 out]
            n217 = call <vilib>:"Error Cluster From Error Code.vi"("show call chain? (False)"=TRUE, "error message (\"\")"=w470, "error code (0)"=5001) -> ("error out"=w476:errorcluster)  [unwired: 6 in]
            n218 = Merge Errors(w478, w476) -> (w477:errorcluster)
          }
          frame "Exit" {
            w486 = 91  # 91: not all Exit messages will have an argument
            w487 = TRUE  # Stop the VI
            # "Release the message queue reference"
            # "#DQMH_CodeNeeded - Add any required cleanup code here."
            # "Exit - Exit the application."
            n219 = Variant To Data(error in=w495, type=T4 {"Module ID"=-1, "Origin"="", "Exit via Stop Module Req?"=FALSE, "Wait for Module to stop?"=FALSE} ("Stop Argument"), Variant=w485) -> (data=w482:T4, error out=w491:errorcluster)
            n220 = call <vilib>:"Clear Errors.vi"("error in (no error)"=w491, "specific error code to clear (0: all)"=w486) -> ("error out"=w494:errorcluster)  [unwired: 4 in, 1 out]
            n221 = property on="Property Node" class="Mod Admin"(reference=w480) -> ("Accessors:Module ID"=w479:i32)  [unwired: 1 in, 2 out]
            n222 = control-ref of="This VI"() -> (w481:refnum<vi>)
            n223 = call-dynamic "Delacor_lib_QMH_Release Message Queue.vi"("error in"=w494, "Message Queue"=w489) -> ("error out"=w493:errorcluster)  [unwired: 9 in]
            n224 = call "Handle Exit.vi"("Stop Argument"=w482, "Module Admin in"=w480, "VI reference"=w481) -> ("error out"=w492:errorcluster, "Wait for Stop?"=w483:bool)  [unwired: 7 in]
            n225 = Merge Errors(w493, w492) -> (w490:errorcluster)
            n226 = call "Error Reported.vi"("Error"=w490, "Module ID"=w479) -> ()  [unwired: 9 in, 1 out]
          }
          frame Default {
            # "'Default' case only runs if there is a message that isn't defined in any of the other cases.  Output a programming error."
            n227 = property on="Property Node" class="Mod Admin"(reference=w503) -> ("Accessors:Module ID"=w502:i32)  [unwired: 1 in, 2 out]
            n228 = call "Module Name--constant.vi"("Module ID"=w502) -> ("Module Name"=w496:string)  [unwired: 10 in]
            n229 = Format Into String(format string="The invalid message string \"%s\" was received in the Message Handling Loop for module \"%s\".", w497, w496) -> (resulting string=w499:string)  [unwired: 2 in, 1 out]
            n230 = call <vilib>:"Error Cluster From Error Code.vi"("show call chain? (False)"=TRUE, "error message (\"\")"=w499, "error code (0)"=1) -> ("error out"=w505:errorcluster)  [unwired: 6 in]
            n231 = Merge Errors(w506, w505) -> (w507:errorcluster)
          }
        }
        n232 = call-dynamic "Delacor_lib_QMH_Error Handler - Message Handling Loop.vi"("error in"=w241, "Message Queue in"=w232) -> ("dup error in"=w238:errorcluster)  [unwired: 8 in, 1 out]
      }
    }
    frame Error {
      n233 = call "Synchronize Caller Events.vi"("Module Admin"=w511) -> ("Module Admin out"=w510:refnum<class "Delacor_lib_QMH_Cloneable Module Admin.lvclass">)  [unwired: 9 in, 1 out]
      n234 = property on="Property Node" class="Mod Admin"(reference=w510) -> ("Accessors:Module ID"=w509:i32)  [unwired: 1 in, 2 out]
      n235 = call-dynamic "Delacor_lib_QMH_Release Message Queue.vi"("error in"=w517, "Message Queue"=w508) -> ("error out"=w516:errorcluster)  [unwired: 9 in]
      n236 = call "Module Name--constant.vi"("Module ID"=w509) -> ("Module Name"=w514:string)  [unwired: 10 in]
      n237 = Format Into String(format string="An error occurred during initialization. %s is no longer running.", w514) -> (resulting string=w512:string)  [unwired: 2 in, 1 out]
      n238 = call "Error Reported.vi"("Additional Information"=w512, "Error"=w516, "Module ID"=w509) -> ()  [unwired: 8 in, 1 out]
    }
  }
  n239 = Merge Errors(w17, w16) -> (w18:errorcluster)
  n240 = call "Close Module.vi"("error in"=w18, "Wait for stop?"=w2, "Module Admin in"=w4) -> ("error out"=w14:errorcluster, "External Launch"=w1:bool, "Module Admin out"=w3:refnum<class "Delacor_lib_QMH_Cloneable Module Admin.lvclass">)  [unwired: 6 in]
  n241 = Unregister For Events(event registration refnum=w9, error in=w14) -> (error out=w13:errorcluster)
  "error out" <- w13
  n242 = case "External Launch?" shown="True" w1 {
    tunnel: w13 -> [_ w518]
    frame False {
    }
    frame True {
      n243 = case shown="No Error" w518 {
        frame No Error {
          n244 = invoke class="VI" method="FP.Close"() -> ()  [unwired: 3 in, 3 out]
        }
        frame Error {
          n245 = disable-structure shown="Default" {
            frame condition #0 (active) {
              n246 = invoke class="VI" method="FP.Open"("Activate"=TRUE ("Activate?")) -> ()  [unwired: 4 in, 5 out]
            }
            frame condition #1 {
              # "Don't show panel on error if running inside a built EXE."
            }
          }
        }
      }
    }
  }
  n247 = local write "Module Admin"(w3) -> ()
